vi "LUT.CreateEntryForDynamicChannels.vi"(8 "error in":errorcluster, 9 "Groups":T1(array[cluster]), 10 "LUT in":variant) -> (0 "error out":errorcluster, 2 "LUT out":variant)   [LabVIEW 2023, in "Data Access Engine.lvlib" / "Data Access Engine.lvclass"]
uses:
  Data Access Engine.lvclass
  Data Access Engine.lvclass/Data Access Engine.ctl
  <vilib>/Utility/Data Type/NI_Data Type.lvlib
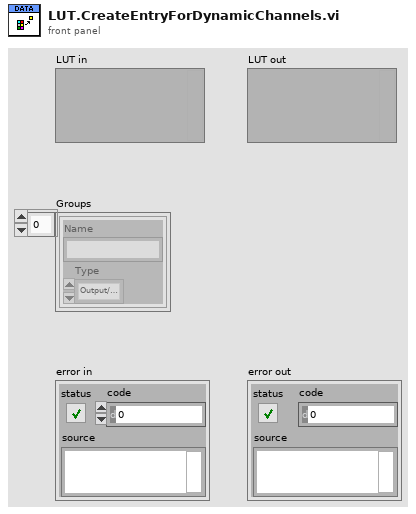
[diagram p1: front panel]
types:
  T1 = cluster{"Name":string, "Type":enum16{"Output/Write", "Input/Read", "Input/ReadWrite"}}[]
  T2 = enum16{"Output/Write", "Input/Read", "Input/ReadWrite"}
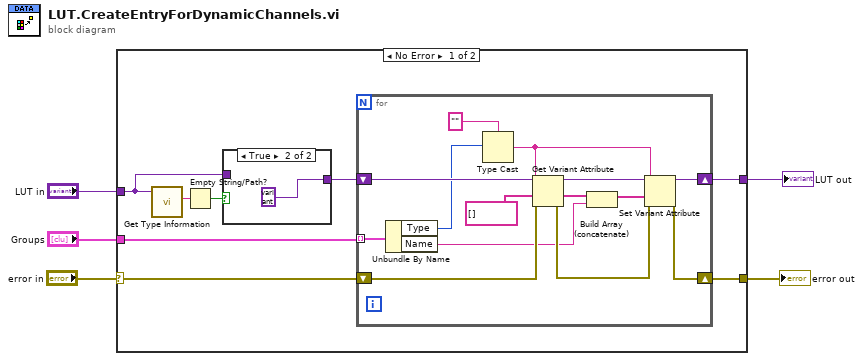
[diagram p0: block diagram]
diagram:
  n1 = case shown="No Error" "error in" {
    selector: "error in" -> [w12 w31]
    tunnel: [w13 w31] -> w5
    tunnel: [w11 w30] -> w3
    tunnel: "Groups" -> [w10 _]
    tunnel: "LUT in" -> [w6 w30]
    frame No Error {
      n2 = call <vilib>:"Get Type Information.vi"("variant"=w6) -> ("name"=w9:string)  [unwired: 6 in, 4 out]
      n3 = Empty String/Path?(string/path=w9) -> (empty?=w8:bool)
      n4 = case shown="True" w8 {
        tunnel: [w14 variant] -> w7
        tunnel: w6 -> [w14 _]
        frame False {
        }
        frame True {
        }
      }
      n5 = for {
        shift-right: [w29] -> w13
        shift-left: w12 -> [w28]
        shift-right: [w22] -> w11
        shift-left: w7 -> [w21]
        tunnel: w10 -> [w19] mode=indexing
        n6 = Unbundle By Name(w19) -> ("Type"=w17:T2, "Name"=w18:string)
        n7 = Type Cast(type="", x=w17) -> (*(type *) &x=w23:string)
        n8 = Get Variant Attribute(Variant=w21, name=w23, default value (empty Variant)=string[] [], error in=w28) -> (duplicate Variant=w20:variant, value=w25:string[], error out=w27:errorcluster)  [unwired: 1 out]
        n9 = Build Array (concatenate)(w25, w18) -> (w26:string[])
        n10 = Set Variant Attribute(Variant=w20, name=w23, value=w26, error in=w27) -> (Variant out=w22:variant, error out=w29:errorcluster)  [unwired: 1 out]
      }
    }
    frame Error {
    }
  }
  "error out" <- w5
  "LUT out" <- w3
